vi "Get Is OperationMode Supported.vi"(8 "error in (no error)":errorcluster, 10 "Operation Mode":i32(ring) items=["SoftwareTriggered", "HardwareTriggered", "Bulb", "Reserved1", "Reserved2"], 11 "TLCamera reference":refnum<k24>) -> (0 "error out":errorcluster, 2 "Is OperationMode Supported":bool, 3 "TLCamera reference out":refnum<k24>)   [LabVIEW 2015]
uses:
  C:/code/ScientificCameraInterfaces/Installer/Scientific Camera Interfaces/LabVIEW/64_bit/Library_X64/Thorlabs.TSI.TLCameraInterfaces.dll
  code/ScientificCameraInterfaces/Installer/Scientific Camera Interfaces/LabVIEW/64_bit/Library_X64/Thorlabs.TSI.TLCameraInterfaces.dll
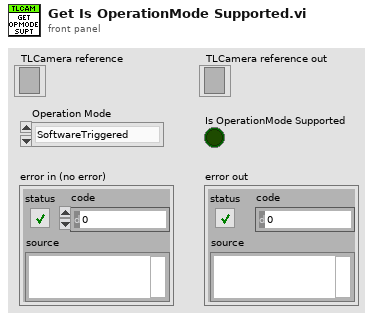
[diagram p1: front panel]
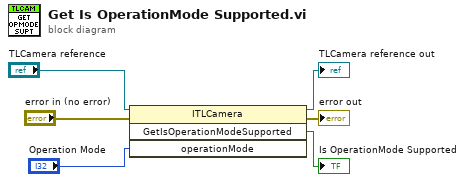
[diagram p0: block diagram]
diagram:
  n1 = invoke class="ITLCamera" method="GetIsOperationModeSupported"(reference="TLCamera reference", error in="error in (no error)", "operationMode"="Operation Mode") -> (reference out=→"TLCamera reference out":refnum<k24>, error out=→"error out":errorcluster, "GetIsOperationModeSupported"=→"Is OperationMode Supported":bool)  [unwired: 1 in, 1 out]
